vi "Refresh Resources.vi"(8 "error in (no error)":errorcluster, 11 "AbstractResourceEnumerator in":refnum<class "AbstractResourceEnumerator.lvclass">) -> (0 "error out":errorcluster, 3 "AbstractResourceEnumerator out":refnum<class "AbstractResourceEnumerator.lvclass">)   [LabVIEW 2023, in "HAF.lvlib" / "AbstractResourceEnumerator.lvclass"]
doc: "Rebuilds the collection of enumerated resources connected to the system."
uses:
  AbstractResourceEnumerator.lvclass
  AbstractResourceEnumerator.lvclass/AbstractResourceEnumerator.ctl
  Resource Structure.ctl
  HAF.lvlib
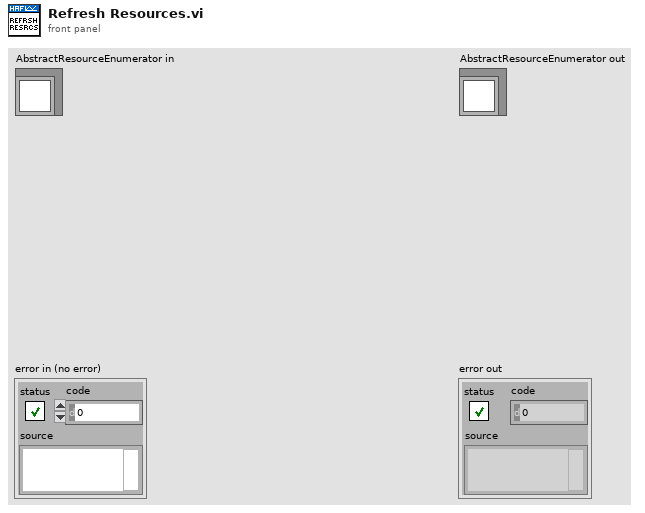
[diagram p1: front panel]
types:
  T1 = typedef "HAF.lvlib/Resource Structure.ctl" = cluster{"Alias":string, "Canonical Name":string}
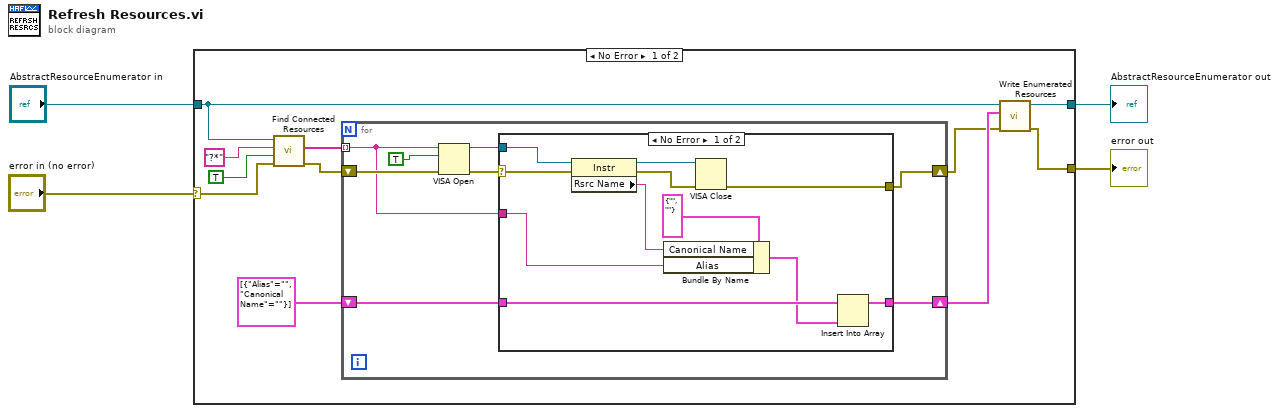
[diagram p0: block diagram]
diagram:
  n1 = case shown="No Error" "error in (no error)" {
    selector: "error in (no error)" -> [w13 w38]
    tunnel: [w5 w38] -> w1
    tunnel: [w6 w37] -> w2
    tunnel: "AbstractResourceEnumerator in" -> [w9 w37]
    frame No Error {
      n2 = call-dynamic "Find Connected Resources.vi"("error in (no error)"=w13, "Return Aliases"=TRUE, "Search Expression"="?*", "AbstractResourceEnumerator in"=w9) -> ("error out"=w11:errorcluster, "Found Resources"=w12:string[])  [unwired: 5 in, 1 out]
      n3 = for {
        tunnel: w12 -> [w19] mode=indexing
        shift-right: [w16] -> w7
        shift-left: w11 -> [w22]
        shift-right: [w17] -> w8
        shift-left: T1[] [{"Alias"="", "Canonical Name"=""}] -> [w18]
        n4 = VISA Open(duplicate session (F)=TRUE, error in (no error)=w22, VISA resource name=w19) -> (VISA resource name=w20:refnum<visa-resource-name>, error out=w21:errorcluster)  [unwired: 2 in]
        n5 = case shown="No Error" w21 {
          selector: w21 -> [w33 w36]
          tunnel: w20 -> [w34 _]
          tunnel: w19 -> [w31 _]
          tunnel: [w27 w36] -> w16
          tunnel: w18 -> [w26 w35]
          tunnel: [w24 w35] -> w17
          frame No Error {
            n6 = property class="Instr"(reference=w34, error in=w33) -> (reference out=w29:refnum<visa-resource-name>, error out=w28:errorcluster, "Rsrc Name"=w30:string)
            n7 = Bundle By Name(cluster=T1 {"Alias"="", "Canonical Name"=""} ("Resource Summary"), "Canonical Name"=w30, "Alias"=w31) -> (w25:T1)
            n8 = VISA Close(VISA resource name=w29, error in (no error)=w28) -> (error out=w27:errorcluster)
            n9 = Insert Into Array(array=w26, new element=w25) -> (w24:T1[])  [unwired: 1 in]
          }
          frame Error {
          }
        }
      }
      n10 = call-dynamic "Write Enumerated Resources.vi"("error in (no error)"=w7, "Enumerated Resources"=w8, "AbstractResourceEnumerator in"=w9) -> ("error out"=w5:errorcluster, "AbstractResourceEnumerator out"=w6:refnum<class "AbstractResourceEnumerator.lvclass">)  [unwired: 7 in]
    }
    frame Error {
    }
  }
  "error out" <- w1
  "AbstractResourceEnumerator out" <- w2
